vi "TSPopup.Make Popup Visible.vi"(6 "LV Version":string, 7 "Popup Parameters":T1, 8 "error in (no error)":errorcluster, 9 "Ctl Offsets":cluster{"Left":i32, "Top":i32}[](array[cluster]), 11 "Popup Cluster Ref":refnum<vi>) -> (0 "error out":errorcluster, 2 "event data":T3)   [LabVIEW 2016, in "TSPopup.lvlib" / "TSPopup.lvclass"]
doc: "Handles all the positioning and setup code to show the proper popup control.\n\nType Sensitive Popup \nCopyright © 2007, J. David Saunders\nAll rights reserved."
uses:
  <userlib>/TSPopup/TSPopup.lvclass
  <userlib>/TSPopup/Private/TSPopup.Monitor Register Data.ctl
  <userlib>/TSPopup/Private/TSPopup.Event Enum.ctl
  <userlib>/TSPopup/TSPopup.Popup Call Parameters.ctl
  <userlib>/TSPopup/TSPopup.Data Type.ctl
panel:
  # "Type Sensitive Popup \nCopyright © 2007, J. David Saunders\nAll rights reserved."
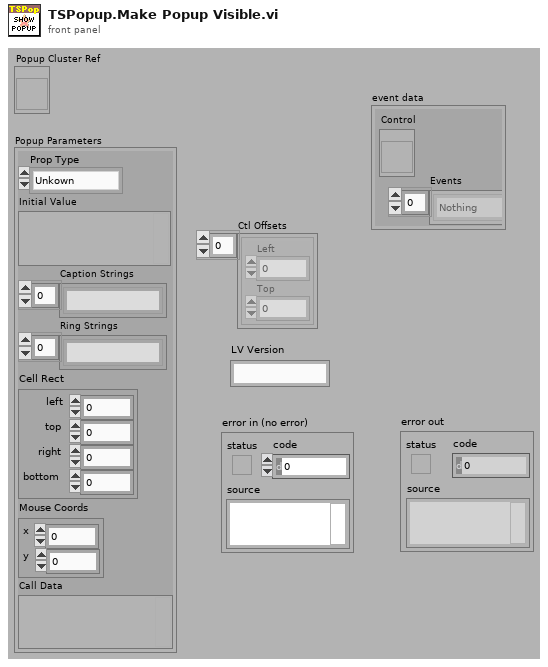
[diagram p1: front panel]
types:
  T1 = typedef "TSPopup.lvlib/TSPopup.lvclass/TSPopup.Popup Call Parameters.ctl" = cluster{"Prop Type":T2, "Initial Value":variant, "Caption Strings":string[], "Ring Strings":string[], "Cell Rect":cluster{"left":i16, "top":i16, "right":i16, "bottom":i16}, "Mouse Coords":cluster{"x":i16, "y":i16}, "Call Data":variant}
  T2 = typedef "TSPopup.lvlib/TSPopup.lvclass/TSPopup.Data Type.ctl" = enum16{"Unkown", "NO POPUP", "String", "Integer", "Float", "Color", "Boolean", "Ring", "Captioned String", "Captioned Integer", "Button Color", "2 Int Cluster", "4 Int Cluster", "check"}
  T3 = typedef "TSPopup.lvlib/TSPopup.lvclass/TSPopup.Monitor Register Data.ctl" = cluster{"Control":refnum<vi>, "Events":T4[]}
  T4 = typedef "TSPopup.lvlib/TSPopup.lvclass/TSPopup.Event Enum.ctl" = enum16{"Nothing", "Enter Key Accept", "Escape Key Cancel", "Mouse Outside Accept", "Mouse Outside Cancel", "Mouse Move Accept", "Mouse Move Cancel", "Mouse Leave Cancel", "Value Change Accept", "Lose Focus Cancel", "Cancel Button", "Accept Button"}
  T5 = cluster{"left":i32, "top":i32, "right":i32, "bottom":i32}
  T6 = cluster{"left":i16, "top":i16, "right":i16, "bottom":i16}
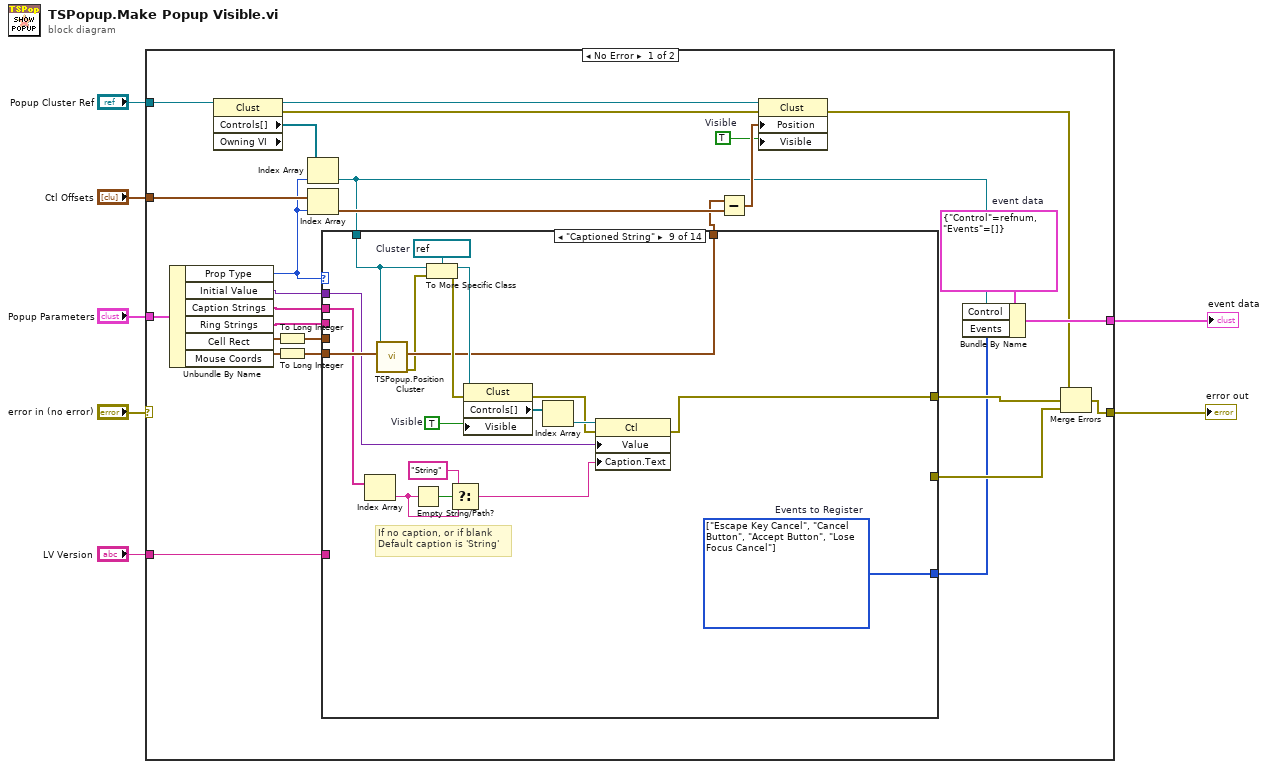
[diagram p0: block diagram]
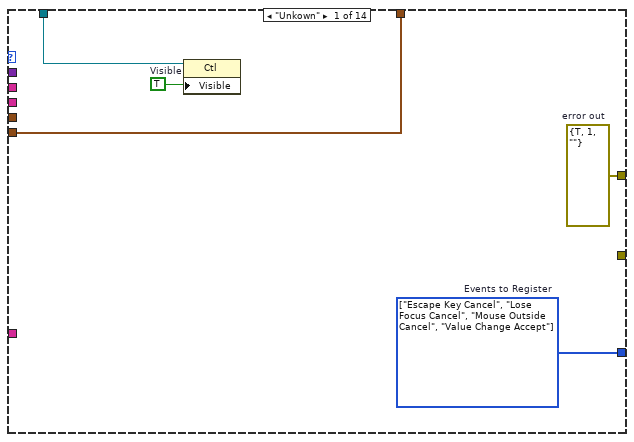
[diagram p2: hidden frame]
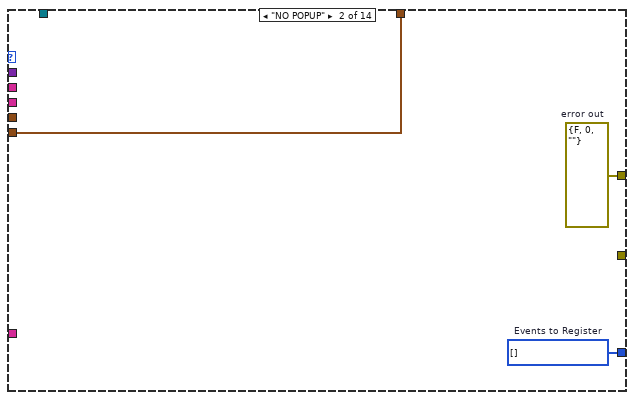
[diagram p3: hidden frame]
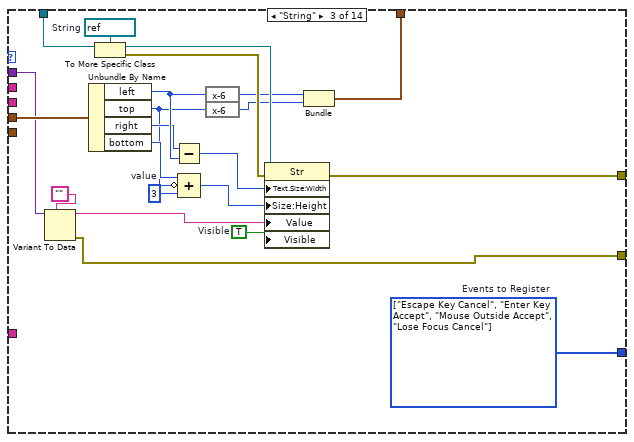
[diagram p4: hidden frame]
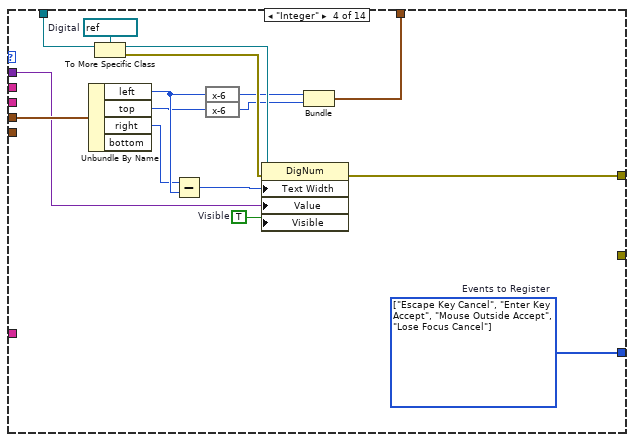
[diagram p5: hidden frame]
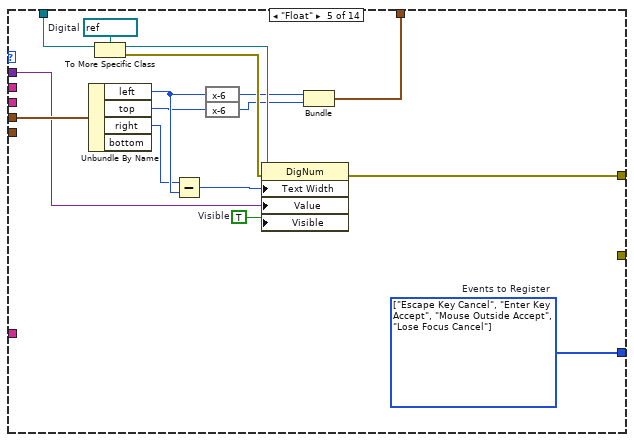
[diagram p6: hidden frame]
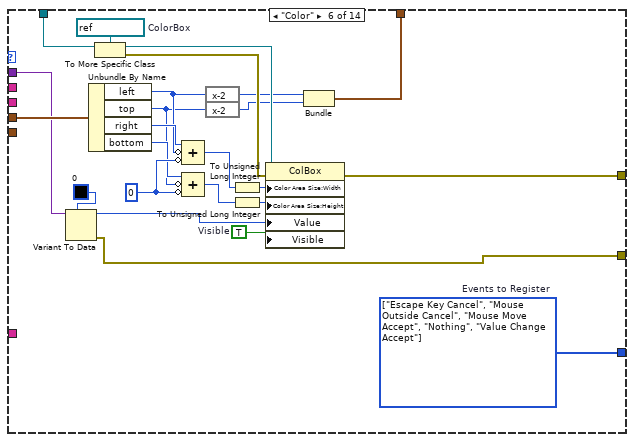
[diagram p7: hidden frame]
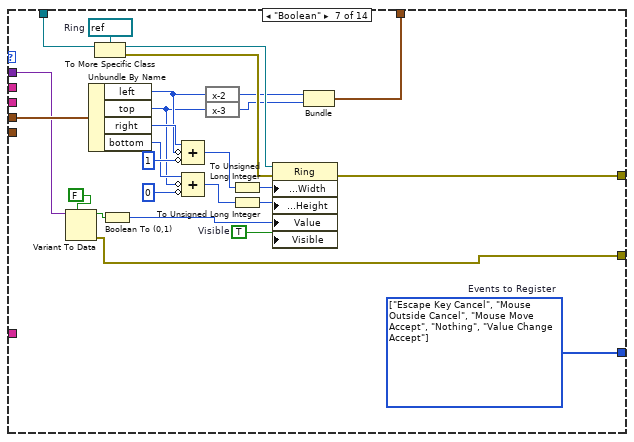
[diagram p8: hidden frame]
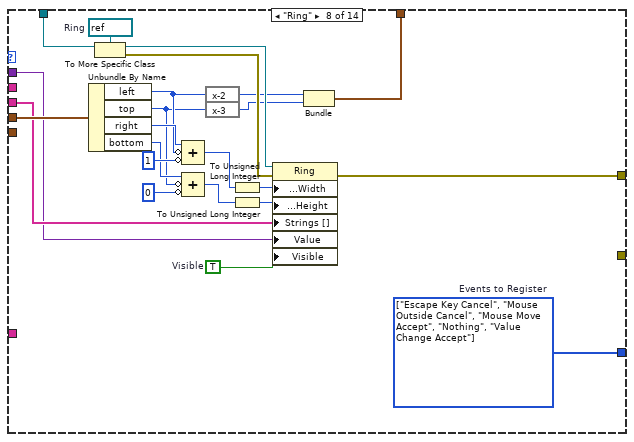
[diagram p9: hidden frame]
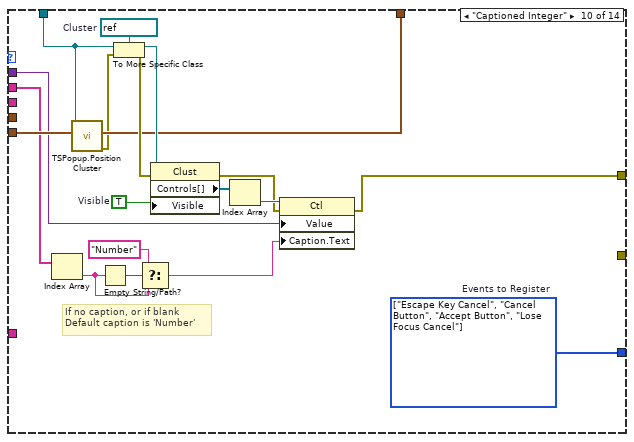
[diagram p10: hidden frame]
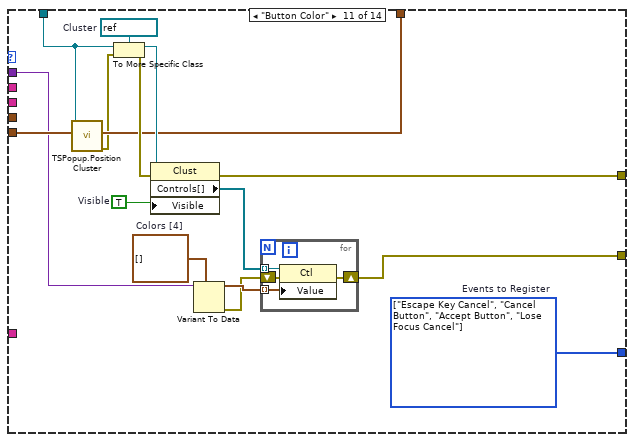
[diagram p11: hidden frame]
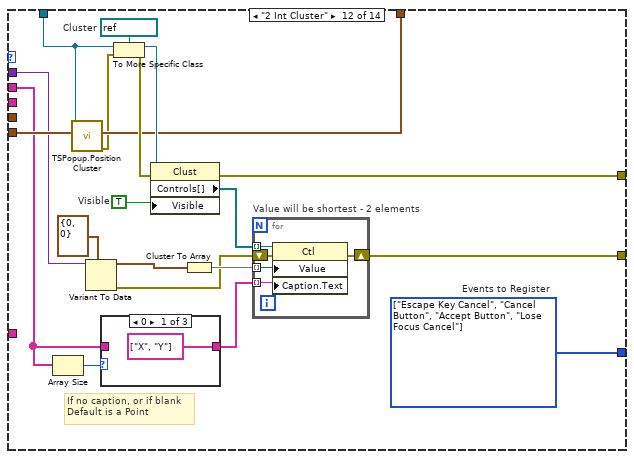
[diagram p12: hidden frame]
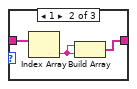
[diagram p13: hidden frame]
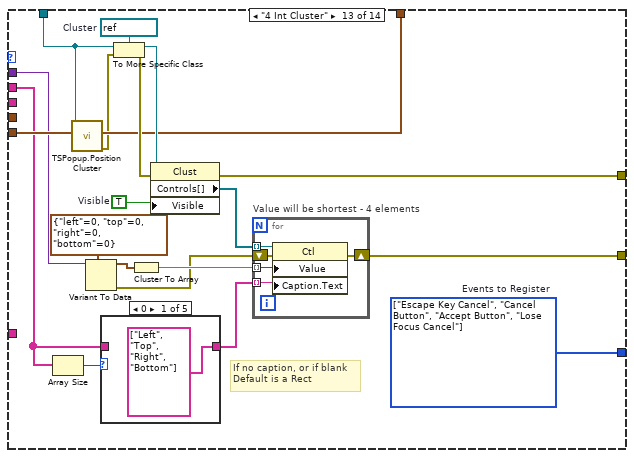
[diagram p15: hidden frame]
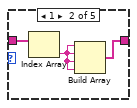
[diagram p16: hidden frame]
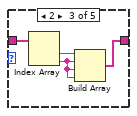
[diagram p17: hidden frame]
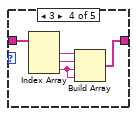
[diagram p18: hidden frame]
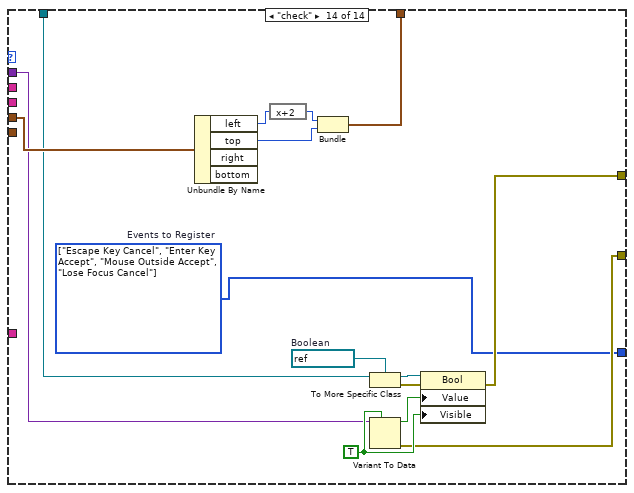
[diagram p20: hidden frame]
diagram:
  n1 = case shown="No Error" "error in (no error)" {
    selector: "error in (no error)" -> [_ w313]
    tunnel: "Popup Parameters" -> [w34 _]
    tunnel: "Popup Cluster Ref" -> [w33 _]
    tunnel: "Ctl Offsets" -> [w31 _]
    tunnel: [w24 w312] -> w4
    tunnel: [w21 w313] -> w2
    tunnel: "LV Version" -> [w13 _]
    frame No Error {
      w30 = T3 {"Control"=refnum, "Events"=[]}  # event data
      w25 = TRUE  # Visible
      n2 = Unbundle By Name(w34) -> ("Prop Type"=w8:T2, "Initial Value"=w18:variant, "Caption Strings"=w17:string[], "Ring Strings"=w16:string[], "Cell Rect"=w28:T6, "Mouse Coords"=w20:cluster{"x":i16, "y":i16})
      n3 = property class="Clust" props=["Controls[]", "Owning VI"](reference=w33) -> (reference out=w29:refnum<vi>, error out=w23:errorcluster, "Controls[]"=w32:refnum<vi>[])  [unwired: 1 in, 1 out]
      n4 = To Long Integer(number=w28) -> (32bit integer=w15:T5)
      n5 = To Long Integer(number=w20) -> (32bit integer=w14:cluster{"x":i32, "y":i32})
      n6 = Index Array(array=w32, index=w8) -> (element=w19:refnum<vi>)
      n7 = Index Array(array=w31, index=w8) -> (element=w27:cluster{"Left":i32, "Top":i32})
      n8 = case shown="\"Captioned String\"" w8 {
        tunnel: w19 -> [w36 _ w54 w76 w92 w118 w144 w167 w178 w197 w215 w239 w269 w303]
        tunnel: w18 -> [_ _ w57 w66 w82 w109 w136 w147 w179 w198 w212 w238 w268 w304]
        tunnel: w15 -> [_ _ w58 w77 w93 w119 w145 w168 _ _ _ _ _ w308]
        tunnel: [w39 w42 w50 w72 w88 w114 w140 w163 w171 w189 w220 w244 w274 w302] -> w11
        tunnel: [w38 w40 w47 w69 w85 w111 w137 w160 w182 w201 w216 w240 w270 w305] -> w9
        tunnel: [w37 w41 w46 w68 w84 w97 w121 w159 w185 w204 w219 w243 w273 w297] -> w10
        tunnel: w16 -> [_ _ _ _ _ _ _ w148 _ _ _ _ _ _]
        tunnel: w14 -> [w38 w40 _ _ _ _ _ _ w183 w202 w217 w241 w271 _]
        tunnel: w17 -> [_ _ _ _ _ _ _ _ w177 w196 _ w236 w266 _]
        tunnel: [_ _ w43 _ _ w98 w122 _ _ _ w208 w232 w258 w301] -> w12
        tunnel: w13 -> [_ _ _ _ _ _ _ _ _ _ _ _ _ _]
        frame "Unkown" {
          w37 = T4[] [enum."Escape Key Cancel", enum."Lose Focus Cancel", enum."Mouse Outside Cancel", enum."Value Change Accept"] items=["Nothing", "Enter Key Accept", "Escape Key Cancel", "Mouse Outside Accept", "Mouse Outside Cancel", "Mouse Move Accept", "Mouse Move Cancel", "Mouse Leave Cancel", "Value Change Accept", "Lose Focus Cancel", "Cancel Button", "Accept Button"]  # Events to Register
          w39 = errorcluster {"status"=TRUE, "code"=1, "source"=""}  # error out
          w35 = TRUE  # Visible
          n9 = property class="Ctl"(reference=w36, "Visible"=w35) -> ()  [unwired: 1 in, 2 out]
        }
        frame "NO POPUP" {
          w41 = T4[] [] items=["Nothing", "Enter Key Accept", "Escape Key Cancel", "Mouse Outside Accept", "Mouse Outside Cancel", "Mouse Move Accept", "Mouse Move Cancel", "Mouse Leave Cancel", "Value Change Accept", "Lose Focus Cancel", "Cancel Button", "Accept Button"]  # Events to Register
          w42 = errorcluster {"status"=FALSE, "code"=0, "source"=""}  # error out
        }
        frame "String" {
          w53 = refnum<vi> refnum  # String
          w59 = TRUE  # Visible
          w60 = 3  # value
          w46 = T4[] [enum."Escape Key Cancel", enum."Enter Key Accept", enum."Mouse Outside Accept", enum."Lose Focus Cancel"] items=["Nothing", "Enter Key Accept", "Escape Key Cancel", "Mouse Outside Accept", "Mouse Outside Cancel", "Mouse Move Accept", "Mouse Move Cancel", "Mouse Leave Cancel", "Value Change Accept", "Lose Focus Cancel", "Cancel Button", "Accept Button"]  # Events to Register
          n10 = Variant To Data(type="", Variant=w57) -> (data=w55:string, error out=w43:errorcluster)  [unwired: 1 in]
          n11 = Unbundle By Name(w58) -> ("left"=w62:i32, "top"=w44:i32, "right"=w45:i32, "bottom"=w64:i32)
          n12 = To More Specific Class(target class=w53, reference=w54) -> (specific class reference=w52:refnum<vi>, error out=w51:errorcluster)  [unwired: 1 in]
          n13 = Subtract(x=w45, y=w62) -> (x-y=w61:i32)
          n14 = Compound Arithmetic op=ADD(w64, invert w44, w60) -> (w63:i32)
          n15 = expression code="x-6"(w62) -> (w49:i32)
          n16 = expression code="x-6"(w44) -> (w48:i32)
          n17 = property class="Str"(reference=w52, error in=w51, "Text.Size:Width"=w61, "Size:Height"=w63, "Value"=w55, "Visible"=w59) -> (error out=w50:errorcluster)  [unwired: 1 out]
          n18 = Bundle("left"=w49, "top"=w48) -> (w47:cluster{"left":i32, "top":i32})  [unwired: 1 in]
        }
        frame "Integer" {
          w75 = refnum<vi> refnum  # Digital
          w78 = TRUE  # Visible
          w68 = T4[] [enum."Escape Key Cancel", enum."Enter Key Accept", enum."Mouse Outside Accept", enum."Lose Focus Cancel"] items=["Nothing", "Enter Key Accept", "Escape Key Cancel", "Mouse Outside Accept", "Mouse Outside Cancel", "Mouse Move Accept", "Mouse Move Cancel", "Mouse Leave Cancel", "Value Change Accept", "Lose Focus Cancel", "Cancel Button", "Accept Button"]  # Events to Register
          n19 = Unbundle By Name(w77) -> ("left"=w80:i32, "top"=w65:i32, "right"=w67:i32)  [unwired: 1 out]
          n20 = To More Specific Class(target class=w75, reference=w76) -> (specific class reference=w74:refnum<vi>, error out=w73:errorcluster)  [unwired: 1 in]
          n21 = Subtract(x=w67, y=w80) -> (x-y=w79:i32)
          n22 = expression code="x-6"(w80) -> (w71:i32)
          n23 = expression code="x-6"(w65) -> (w70:i32)
          n24 = property class="DigNum"(reference=w74, error in=w73, "Text Width"=w79, "Value"=w66, "Visible"=w78) -> (error out=w72:errorcluster)  [unwired: 1 out]
          n25 = Bundle("left"=w71, "top"=w70) -> (w69:cluster{"left":i32, "top":i32})  [unwired: 1 in]
        }
        frame "Float" {
          w91 = refnum<vi> refnum  # Digital
          w94 = TRUE  # Visible
          w84 = T4[] [enum."Escape Key Cancel", enum."Enter Key Accept", enum."Mouse Outside Accept", enum."Lose Focus Cancel"] items=["Nothing", "Enter Key Accept", "Escape Key Cancel", "Mouse Outside Accept", "Mouse Outside Cancel", "Mouse Move Accept", "Mouse Move Cancel", "Mouse Leave Cancel", "Value Change Accept", "Lose Focus Cancel", "Cancel Button", "Accept Button"]  # Events to Register
          n26 = Unbundle By Name(w93) -> ("left"=w96:i32, "top"=w81:i32, "right"=w83:i32)  [unwired: 1 out]
          n27 = To More Specific Class(target class=w91, reference=w92) -> (specific class reference=w90:refnum<vi>, error out=w89:errorcluster)  [unwired: 1 in]
          n28 = Subtract(x=w83, y=w96) -> (x-y=w95:i32)
          n29 = expression code="x-6"(w96) -> (w87:i32)
          n30 = expression code="x-6"(w81) -> (w86:i32)
          n31 = property class="DigNum"(reference=w90, error in=w89, "Text Width"=w95, "Value"=w82, "Visible"=w94) -> (error out=w88:errorcluster)  [unwired: 1 out]
          n32 = Bundle("left"=w87, "top"=w86) -> (w85:cluster{"left":i32, "top":i32})  [unwired: 1 in]
        }
        frame "Color" {
          w97 = T4[] [enum."Escape Key Cancel", enum."Mouse Outside Cancel", enum."Mouse Move Accept", enum."Nothing", enum."Value Change Accept"] items=["Nothing", "Enter Key Accept", "Escape Key Cancel", "Mouse Outside Accept", "Mouse Outside Cancel", "Mouse Move Accept", "Mouse Move Cancel", "Mouse Leave Cancel", "Value Change Accept", "Lose Focus Cancel", "Cancel Button", "Accept Button"]  # Events to Register
          w117 = refnum<vi> refnum  # ColorBox
          w107 = 0
          w120 = TRUE  # Visible
          n33 = Variant To Data(type=u32 0, Variant=w109) -> (data=w108:u32, error out=w98:errorcluster)  [unwired: 1 in]
          n34 = Unbundle By Name(w119) -> ("left"=w105:i32, "top"=w103:i32, "right"=w106:i32, "bottom"=w104:i32)
          n35 = To More Specific Class(target class=w117, reference=w118) -> (specific class reference=w116:refnum<vi>, error out=w115:errorcluster)  [unwired: 1 in]
          n36 = Compound Arithmetic op=ADD(w106, invert w105, invert w107) -> (w101:i32)
          n37 = Compound Arithmetic op=ADD(w104, invert w103, invert w107) -> (w102:i32)
          n38 = expression code="x-2"(w105) -> (w113:i32)
          n39 = expression code="x-2"(w103) -> (w112:i32)
          n40 = To Unsigned Long Integer(number=w101) -> (unsigned 32bit integer=w100:u32)
          n41 = To Unsigned Long Integer(number=w102) -> (unsigned 32bit integer=w99:u32)
          n42 = property class="ColBox"(reference=w116, error in=w115, "Color Area Size:Width"=w100, "Color Area Size:Height"=w99, "Value"=w108, "Visible"=w120) -> (error out=w114:errorcluster)  [unwired: 1 out]
          n43 = Bundle("left"=w113, "top"=w112) -> (w111:cluster{"left":i32, "top":i32})  [unwired: 1 in]
        }
        frame "Boolean" {
          w121 = T4[] [enum."Escape Key Cancel", enum."Mouse Outside Cancel", enum."Mouse Move Accept", enum."Nothing", enum."Value Change Accept"] items=["Nothing", "Enter Key Accept", "Escape Key Cancel", "Mouse Outside Accept", "Mouse Outside Cancel", "Mouse Move Accept", "Mouse Move Cancel", "Mouse Leave Cancel", "Value Change Accept", "Lose Focus Cancel", "Cancel Button", "Accept Button"]  # Events to Register
          w143 = refnum<vi> refnum  # Ring
          w146 = TRUE  # Visible
          n44 = Variant To Data(type=FALSE, Variant=w136) -> (data=w135:bool, error out=w122:errorcluster)  [unwired: 1 in]
          n45 = Unbundle By Name(w145) -> ("left"=w132:i32, "top"=w130:i32, "right"=w133:i32, "bottom"=w131:i32)
          n46 = To More Specific Class(target class=w143, reference=w144) -> (specific class reference=w142:refnum<vi>, error out=w141:errorcluster)  [unwired: 1 in]
          n47 = Boolean To (0,1)(Boolean=w135) -> (0, 1=w124:i16)
          n48 = Compound Arithmetic op=ADD(w133, invert w132, invert 1) -> (w128:i32)
          n49 = Compound Arithmetic op=ADD(w131, invert w130, invert 0) -> (w129:i32)
          n50 = expression code="x-2"(w132) -> (w139:i32)
          n51 = expression code="x-3"(w130) -> (w138:i32)
          n52 = To Unsigned Long Integer(number=w128) -> (unsigned 32bit integer=w127:u32)
          n53 = To Unsigned Long Integer(number=w129) -> (unsigned 32bit integer=w126:u32)
          n54 = property class="Ring"(reference=w142, error in=w141, "Named Numeric Size:Width"=w127, "Named Numeric Size:Height"=w126, "Value"=w124, "Visible"=w146) -> (error out=w140:errorcluster)  [unwired: 1 out]
          n55 = Bundle("left"=w139, "top"=w138) -> (w137:cluster{"left":i32, "top":i32})  [unwired: 1 in]
        }
        frame "Ring" {
          w159 = T4[] [enum."Escape Key Cancel", enum."Mouse Outside Cancel", enum."Mouse Move Accept", enum."Nothing", enum."Value Change Accept"] items=["Nothing", "Enter Key Accept", "Escape Key Cancel", "Mouse Outside Accept", "Mouse Outside Cancel", "Mouse Move Accept", "Mouse Move Cancel", "Mouse Leave Cancel", "Value Change Accept", "Lose Focus Cancel", "Cancel Button", "Accept Button"]  # Events to Register
          w166 = refnum<vi> refnum  # Ring
          w169 = TRUE  # Visible
          n56 = Unbundle By Name(w168) -> ("left"=w156:i32, "top"=w154:i32, "right"=w157:i32, "bottom"=w155:i32)
          n57 = To More Specific Class(target class=w166, reference=w167) -> (specific class reference=w165:refnum<vi>, error out=w164:errorcluster)  [unwired: 1 in]
          n58 = Compound Arithmetic op=ADD(w157, invert w156, invert 1) -> (w152:i32)
          n59 = Compound Arithmetic op=ADD(w155, invert w154, invert 0) -> (w153:i32)
          n60 = expression code="x-2"(w156) -> (w162:i32)
          n61 = expression code="x-3"(w154) -> (w161:i32)
          n62 = To Unsigned Long Integer(number=w152) -> (unsigned 32bit integer=w151:u32)
          n63 = To Unsigned Long Integer(number=w153) -> (unsigned 32bit integer=w150:u32)
          n64 = property class="Ring"(reference=w165, error in=w164, "Named Numeric Size:Width"=w151, "Named Numeric Size:Height"=w150, "Strings []"=w148, "Value"=w147, "Visible"=w169) -> (error out=w163:errorcluster)  [unwired: 1 out]
          n65 = Bundle("left"=w162, "top"=w161) -> (w160:cluster{"left":i32, "top":i32})  [unwired: 1 in]
        }
        frame "Captioned String" {
          w188 = refnum<vi> refnum  # Cluster
          w184 = TRUE  # Visible
          w185 = T4[] [enum."Escape Key Cancel", enum."Cancel Button", enum."Accept Button", enum."Lose Focus Cancel"] items=["Nothing", "Enter Key Accept", "Escape Key Cancel", "Mouse Outside Accept", "Mouse Outside Cancel", "Mouse Move Accept", "Mouse Move Cancel", "Mouse Leave Cancel", "Value Change Accept", "Lose Focus Cancel", "Cancel Button", "Accept Button"]  # Events to Register
          # "If no caption, or if blank\nDefault caption is 'String'"
          n66 = Index Array(array=w177) -> (element=w175:string)  [unwired: 1 in]
          n67 = call <userlib>:"TSPopup.Position Cluster.vi"("Mouse Coords"=w183, "Ctl Refnum"=w178) -> ("error out"=w170:errorcluster, "Cluster Pos"=w182:cluster{"x":i32, "y":i32})  [unwired: 7 in, 1 out]
          n68 = Empty String/Path?(string/path=w175) -> (empty?=w176:bool)
          n69 = To More Specific Class(target class=w188, reference=w178, error in=w170) -> (specific class reference=w187:refnum<vi>, error out=w186:errorcluster)
          n70 = Select(t="String", s=w176, f=w175) -> (s? t:f=w173:string)
          n71 = property class="Clust"(reference=w187, error in=w186, "Visible"=w184) -> (error out=w172:errorcluster, "Controls[]"=w180:refnum<vi>[])  [unwired: 1 out]
          n72 = Index Array(array=w180) -> (element=w181:refnum<vi>)  [unwired: 1 in]
          n73 = property class="Ctl"(reference=w181, error in=w172, "Value"=w179, "Caption.Text"=w173) -> (error out=w171:errorcluster)  [unwired: 1 out]
        }
        frame "Captioned Integer" {
          w207 = refnum<vi> refnum  # Cluster
          w203 = TRUE  # Visible
          w204 = T4[] [enum."Escape Key Cancel", enum."Cancel Button", enum."Accept Button", enum."Lose Focus Cancel"] items=["Nothing", "Enter Key Accept", "Escape Key Cancel", "Mouse Outside Accept", "Mouse Outside Cancel", "Mouse Move Accept", "Mouse Move Cancel", "Mouse Leave Cancel", "Value Change Accept", "Lose Focus Cancel", "Cancel Button", "Accept Button"]  # Events to Register
          # "If no caption, or if blank\nDefault caption is 'Number'"
          n74 = Index Array(array=w196) -> (element=w194:string)  [unwired: 1 in]
          n75 = call <userlib>:"TSPopup.Position Cluster.vi"("Mouse Coords"=w202, "Ctl Refnum"=w197) -> ("error out"=w191:errorcluster, "Cluster Pos"=w201:cluster{"x":i32, "y":i32})  [unwired: 7 in, 1 out]
          n76 = Empty String/Path?(string/path=w194) -> (empty?=w195:bool)
          n77 = To More Specific Class(target class=w207, reference=w197, error in=w191) -> (specific class reference=w206:refnum<vi>, error out=w205:errorcluster)
          n78 = Select(t="Number", s=w195, f=w194) -> (s? t:f=w192:string)
          n79 = property class="Clust"(reference=w206, error in=w205, "Visible"=w203) -> (error out=w190:errorcluster, "Controls[]"=w199:refnum<vi>[])  [unwired: 1 out]
          n80 = Index Array(array=w199) -> (element=w200:refnum<vi>)  [unwired: 1 in]
          n81 = property class="Ctl"(reference=w200, error in=w190, "Value"=w198, "Caption.Text"=w192) -> (error out=w189:errorcluster)  [unwired: 1 out]
        }
        frame "Button Color" {
          w214 = cluster{u32, u32}[] []  # Colors [4]
          w223 = refnum<vi> refnum  # Cluster
          w218 = TRUE  # Visible
          w219 = T4[] [enum."Escape Key Cancel", enum."Cancel Button", enum."Accept Button", enum."Lose Focus Cancel"] items=["Nothing", "Enter Key Accept", "Escape Key Cancel", "Mouse Outside Accept", "Mouse Outside Cancel", "Mouse Move Accept", "Mouse Move Cancel", "Mouse Leave Cancel", "Value Change Accept", "Lose Focus Cancel", "Cancel Button", "Accept Button"]  # Events to Register
          n82 = call <userlib>:"TSPopup.Position Cluster.vi"("Mouse Coords"=w217, "Ctl Refnum"=w215) -> ("error out"=w210:errorcluster, "Cluster Pos"=w216:cluster{"x":i32, "y":i32})  [unwired: 7 in, 1 out]
          n83 = To More Specific Class(target class=w223, reference=w215, error in=w210) -> (specific class reference=w222:refnum<vi>, error out=w221:errorcluster)
          n84 = property class="Clust"(reference=w222, error in=w221, "Visible"=w218) -> (error out=w220:errorcluster, "Controls[]"=w211:refnum<vi>[])  [unwired: 1 out]
          n85 = Variant To Data(type=w214, Variant=w212) -> (data=w213:cluster{u32, u32}[], error out=w209:errorcluster)  [unwired: 1 in]
          n86 = for {
            tunnel: w213 -> [w226] mode=indexing
            tunnel: w211 -> [w227] mode=indexing
            shift-right: [w224] -> w208
            shift-left: w209 -> [w225]
            n87 = property class="Ctl"(reference=w227, error in=w225, "Value"=w226) -> (error out=w224:errorcluster)  [unwired: 1 out]
          }
        }
        frame "2 Int Cluster" {
          w247 = refnum<vi> refnum  # Cluster
          w242 = TRUE  # Visible
          w243 = T4[] [enum."Escape Key Cancel", enum."Cancel Button", enum."Accept Button", enum."Lose Focus Cancel"] items=["Nothing", "Enter Key Accept", "Escape Key Cancel", "Mouse Outside Accept", "Mouse Outside Cancel", "Mouse Move Accept", "Mouse Move Cancel", "Mouse Leave Cancel", "Value Change Accept", "Lose Focus Cancel", "Cancel Button", "Accept Button"]  # Events to Register
          # "If no caption, or if blank\nDefault is a Point"
          n88 = Array Size(array=w236) -> (size(s)=w237:i32)
          n89 = call <userlib>:"TSPopup.Position Cluster.vi"("Mouse Coords"=w241, "Ctl Refnum"=w239) -> ("error out"=w233:errorcluster, "Cluster Pos"=w240:cluster{"x":i32, "y":i32})  [unwired: 7 in, 1 out]
          n90 = Variant To Data(type=cluster{"X":i32, "Y":i32} {"X"=0, "Y"=0}, Variant=w238) -> (data=w228:cluster{"X":i32, "Y":i32}, error out=w229:errorcluster)  [unwired: 1 in]
          n91 = case shown="0" w237 {
            tunnel: w236 -> [_ w256 w257]
            tunnel: [string[] ["X", "Y"] w254 w257] -> w235
            frame 0 {
            }
            frame 1 {
              n92 = Index Array(array=w256) -> (element=w255:string)  [unwired: 1 in]
              n93 = Build Array(w255, w255) -> (w254:string[])
            }
            frame 2, Default {
            }
          }
          n94 = To More Specific Class(target class=w247, reference=w239, error in=w233) -> (specific class reference=w246:refnum<vi>, error out=w245:errorcluster)
          n95 = property class="Clust"(reference=w246, error in=w245, "Visible"=w242) -> (error out=w244:errorcluster, "Controls[]"=w234:refnum<vi>[])  [unwired: 1 out]
          n96 = Cluster To Array(cluster=w228) -> (array=w230:i32[])
          n97 = for "Value will be shortest - 2 elements" {
            tunnel: w230 -> [w252] mode=indexing
            tunnel: w235 -> [w251] mode=indexing
            tunnel: w234 -> [w250] mode=indexing
            shift-right: [w248] -> w232
            shift-left: w229 -> [w249]
            n98 = property class="Ctl"(reference=w250, error in=w249, "Value"=w252, "Caption.Text"=w251) -> (error out=w248:errorcluster)  [unwired: 1 out]
          }
        }
        frame "4 Int Cluster" {
          w277 = refnum<vi> refnum  # Cluster
          w272 = TRUE  # Visible
          w273 = T4[] [enum."Escape Key Cancel", enum."Cancel Button", enum."Accept Button", enum."Lose Focus Cancel"] items=["Nothing", "Enter Key Accept", "Escape Key Cancel", "Mouse Outside Accept", "Mouse Outside Cancel", "Mouse Move Accept", "Mouse Move Cancel", "Mouse Leave Cancel", "Value Change Accept", "Lose Focus Cancel", "Cancel Button", "Accept Button"]  # Events to Register
          # "If no caption, or if blank\nDefault is a Rect"
          n99 = Array Size(array=w266) -> (size(s)=w267:i32)
          n100 = call <userlib>:"TSPopup.Position Cluster.vi"("Mouse Coords"=w271, "Ctl Refnum"=w269) -> ("error out"=w260:errorcluster, "Cluster Pos"=w270:cluster{"x":i32, "y":i32})  [unwired: 7 in, 1 out]
          n101 = Variant To Data(type=T5 {"left"=0, "top"=0, "right"=0, "bottom"=0} ("rect"), Variant=w268) -> (data=w263:T5, error out=w259:errorcluster)  [unwired: 1 in]
          n102 = case shown="0" w267 {
            tunnel: w266 -> [_ w286 w290 w295 w296]
            tunnel: [string[] ["Left", "Top", "Right", "Bottom"] w285 w289 w294 w296] -> w265
            frame 0 {
            }
            frame 1 {
              n103 = Index Array(array=w286) -> (element=w284:string)  [unwired: 1 in]
              n104 = Build Array(w284, w284, w284, w284) -> (w285:string[])
            }
            frame 2 {
              n105 = Index Array(array=w290) -> (element #1=w288:string, element #2=w287:string)  [unwired: 2 in]
              n106 = Build Array(w288, w287, w287, w287) -> (w289:string[])
            }
            frame 3 {
              n107 = Index Array(array=w295) -> (element #1=w293:string, element #2=w292:string, element #3=w291:string)  [unwired: 3 in]
              n108 = Build Array(w293, w292, w291, w291) -> (w294:string[])
            }
            frame 4, Default {
            }
          }
          n109 = To More Specific Class(target class=w277, reference=w269, error in=w260) -> (specific class reference=w276:refnum<vi>, error out=w275:errorcluster)
          n110 = Cluster To Array(cluster=w263) -> (array=w262:i32[])
          n111 = property class="Clust"(reference=w276, error in=w275, "Visible"=w272) -> (error out=w274:errorcluster, "Controls[]"=w264:refnum<vi>[])  [unwired: 1 out]
          n112 = for "Value will be shortest - 4 elements" {
            tunnel: w262 -> [w282] mode=indexing
            tunnel: w265 -> [w281] mode=indexing
            tunnel: w264 -> [w280] mode=indexing
            shift-right: [w278] -> w258
            shift-left: w259 -> [w279]
            n113 = property class="Ctl"(reference=w280, error in=w279, "Value"=w282, "Caption.Text"=w281) -> (error out=w278:errorcluster)  [unwired: 1 out]
          }
        }
        frame "check" {
          w297 = T4[] [enum."Escape Key Cancel", enum."Enter Key Accept", enum."Mouse Outside Accept", enum."Lose Focus Cancel"] items=["Nothing", "Enter Key Accept", "Escape Key Cancel", "Mouse Outside Accept", "Mouse Outside Cancel", "Mouse Move Accept", "Mouse Move Cancel", "Mouse Leave Cancel", "Value Change Accept", "Lose Focus Cancel", "Cancel Button", "Accept Button"]  # Events to Register
          w306 = TRUE
          w311 = refnum<vi> refnum  # Boolean
          n114 = Unbundle By Name(w308) -> ("left"=w299:i32, "top"=w300:i32)  [unwired: 2 out]
          n115 = expression code="x+2"(w299) -> (w298:i32)
          n116 = Bundle("left"=w298, "top"=w300) -> (w305:cluster{"left":i32, "top":i32})  [unwired: 1 in]
          n117 = To More Specific Class(target class=w311, reference=w303) -> (specific class reference=w310:refnum<vi>, error out=w309:errorcluster)  [unwired: 1 in]
          n118 = Variant To Data(type=w306, Variant=w304) -> (data=w307:bool, error out=w301:errorcluster)  [unwired: 1 in]
          n119 = property class="Bool"(reference=w310, error in=w309, "Value"=w307, "Visible"=w306) -> (error out=w302:errorcluster)  [unwired: 1 out]
        }
      }
      n120 = Subtract(x=w9, y=w27) -> (x-y=w26:cluster{i32, i32})
      n121 = property class="Clust"(reference=w29, error in=w23, "Position"=w26, "Visible"=w25) -> (error out=w22:errorcluster)  [unwired: 1 out]
      n122 = Bundle By Name(cluster=w30, "Control"=w19, "Events"=w10) -> (w24:T3)
      n123 = Merge Errors(w22, w11, w12) -> (w21:errorcluster)
    }
    frame Error {
      w312 = T3 {"Control"=refnum, "Events"=[]}  # event data
    }
  }
  "event data" <- w4
  "error out" <- w2
